vi "IP SNIFFER main vi.vi"() -> ()   [LabVIEW 2011]
doc: "This VI is an application to run through IP addresses starting at a specific IP and counting up by 1 however many times the user specifies."
uses:
  <vilib>/Utility/sysdir.llb/System Directory Type.ctl
panel:
  in  "Current IP":bool
  in  "Limit":bool
  out "Status":bool
  in  "Save results":bool
  out "Ping returns":T1(array[cluster])
  in  "stop scan":bool
  in  "scan":bool
  in  "Start IP Address (192.168.0.100)":string
  in  "Number of IPs to scan":i32 min=0 max=255 step=1
  in  "stop":bool
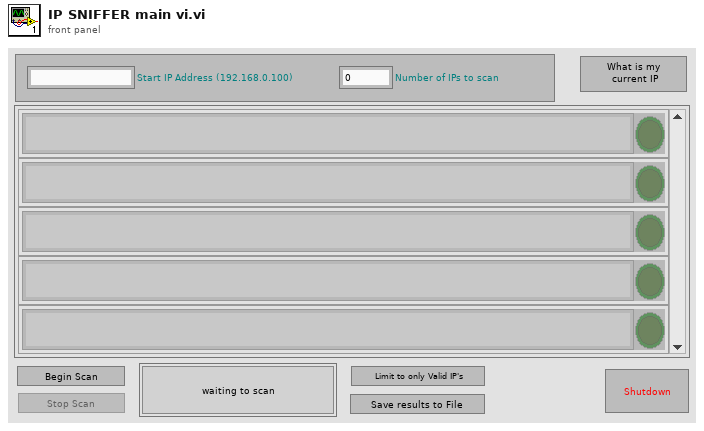
[diagram p1: front panel]
types:
  T1 = cluster{"Ping Status Return":string, "Valid IP (valid = true)":bool}[]
  T2 = cluster{"Ping Status Return":string, "Valid IP (valid = true)":bool}
  T3 = enum16{"open", "replace", "create", "open or create", "replace or create", "replace or create with confirmation"}
  T4 = typedef "System Directory Type.ctl" = i32
  T5 = enum8{"Enabled", "Disabled", "Disabled and Grayed Out"}
  T6 = enum32{"invalid app kind", "Development System", "Run Time System", "Student Edition", "Embedded LabVIEW", "Evaluation", "Custom"}
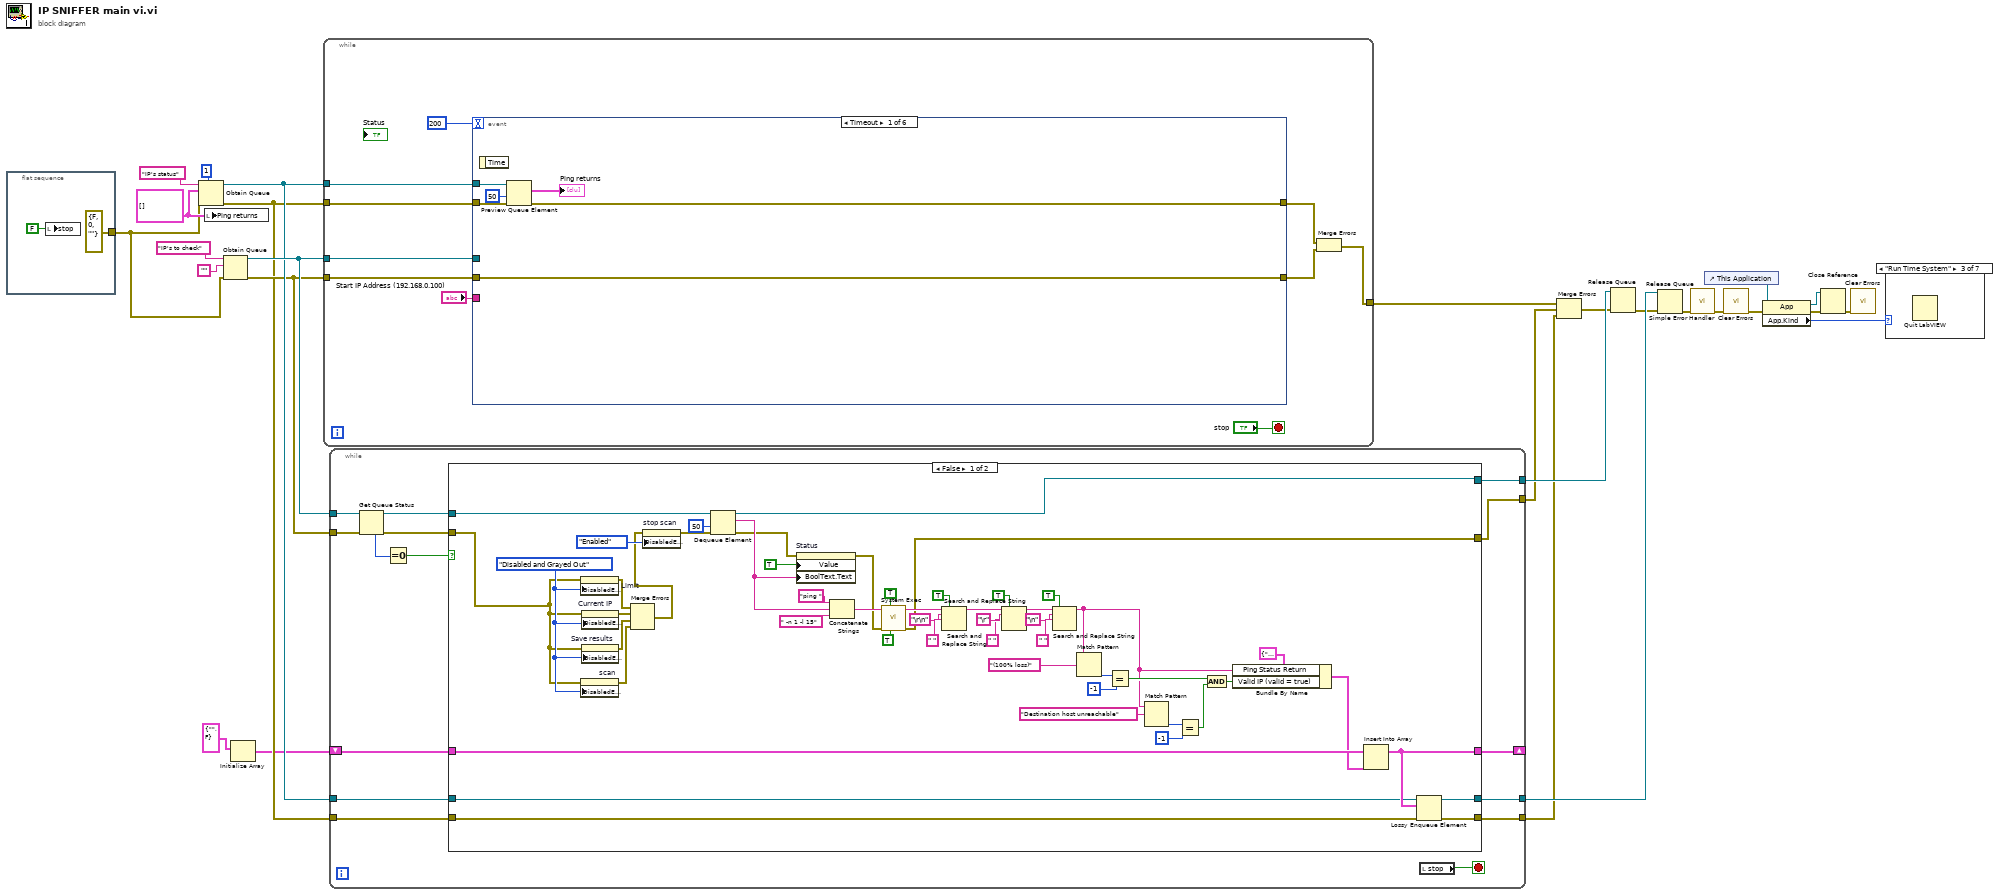
[diagram p0: block diagram]
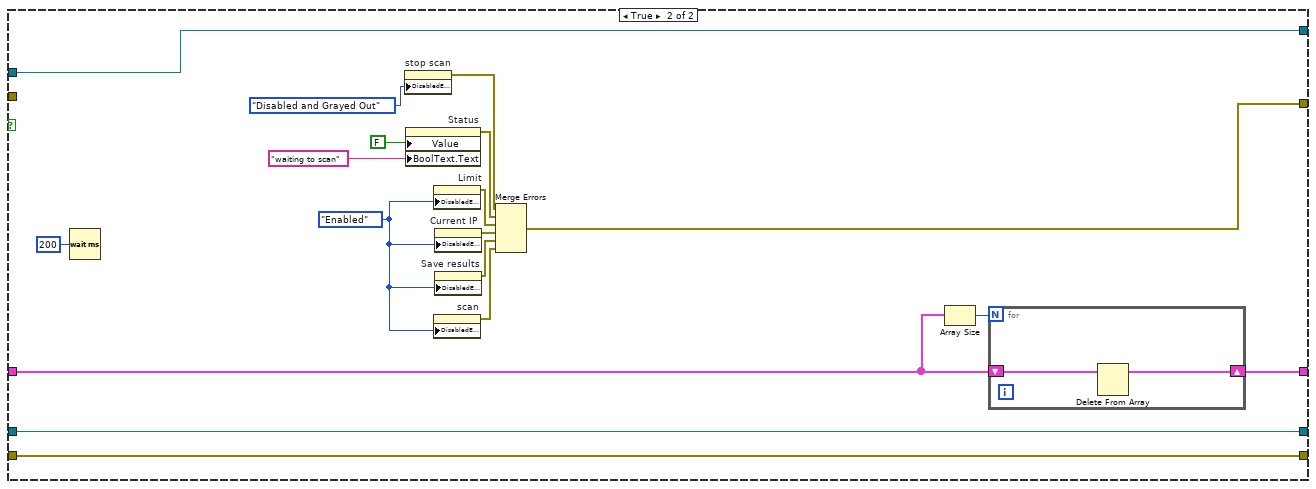
[diagram p2: hidden frame]
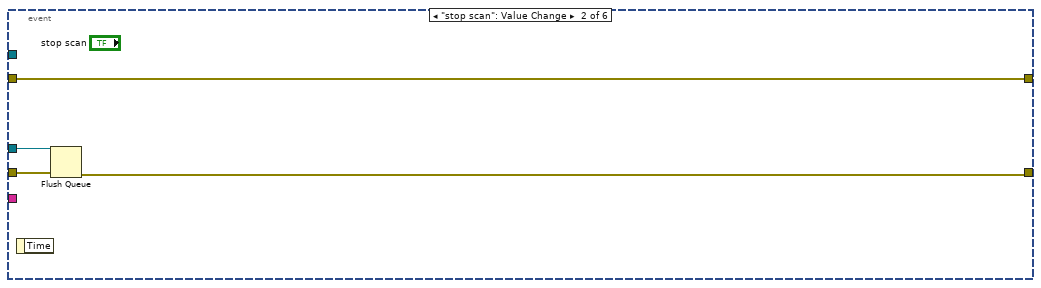
[diagram p9: hidden frame]
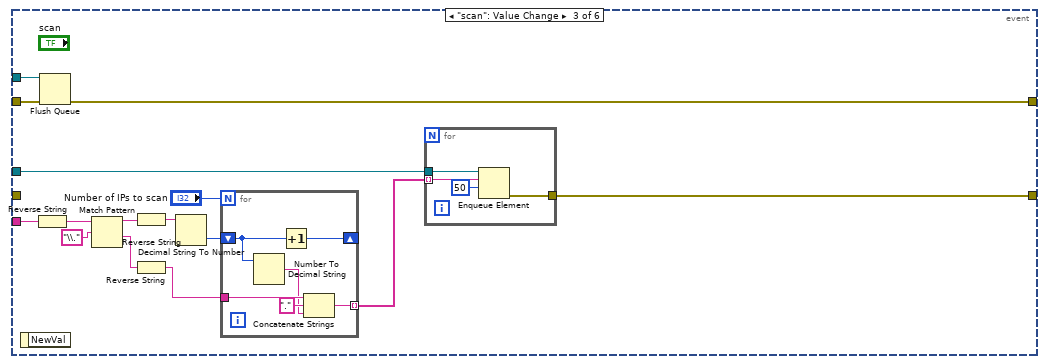
[diagram p10: hidden frame]
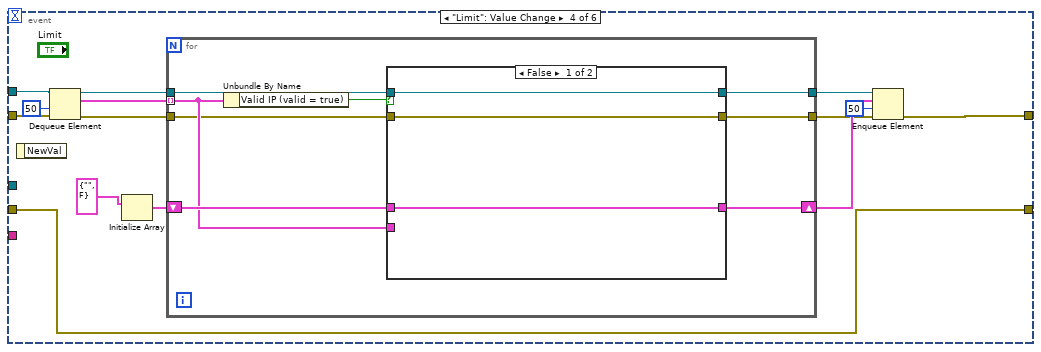
[diagram p11: hidden frame]
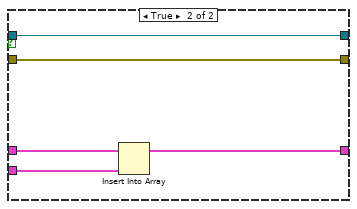
[diagram p12: hidden frame]
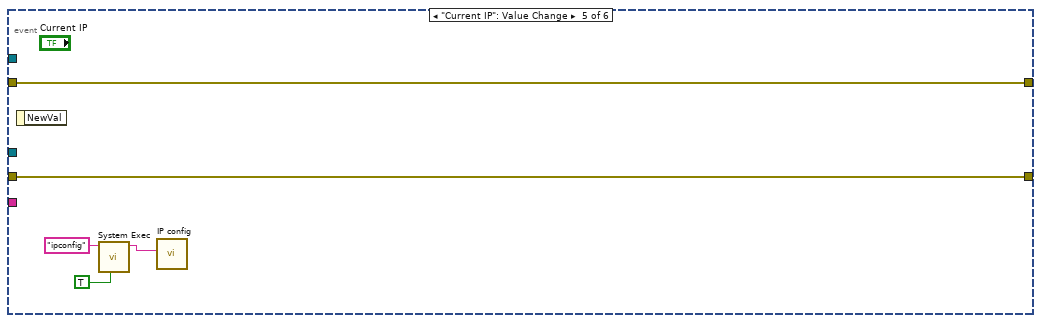
[diagram p13: hidden frame]
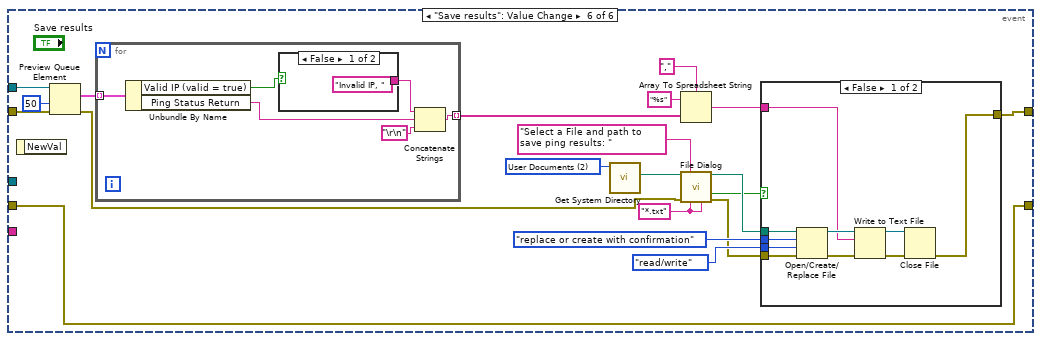
[diagram p14: hidden frame]
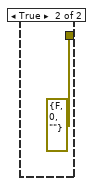
[diagram p15: hidden frame]
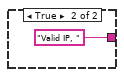
[diagram p16: hidden frame]
diagram:
  w15 = T1 [] ("Ping returns")
  n1 = flat-sequence {
    tunnel: [errorcluster {"status"=FALSE, "code"=0, "source"=""} ("error constant")] -> w6
    frame #0 {
      n2 = local write "stop"(FALSE ("stop")) -> ()
    }
  }
  n3 = Obtain Queue(max queue size (-1, unlimited)=1, name (unnamed)="IP's status", element data type=w15, error in (no error)=w6) -> (queue out=w14:refnum<queue>, error out=w12:errorcluster)  [unwired: 1 in, 1 out]
  n4 = local write "Ping returns"(w15) -> ()
  n5 = Obtain Queue(name (unnamed)="IP's to check", element data type="", error in (no error)=w6) -> (queue out=w19:refnum<queue>, error out=w13:errorcluster)  [unwired: 2 in, 1 out]
  n6 = Initialize Array(T2 {"Ping Status Return"="", "Valid IP (valid = true)"=FALSE}) -> (w10:T1)  [unwired: 1 in]
  n7 = while {
    tunnel: [w30] -> w25
    tunnel: w19 -> [w37]
    tunnel: w14 -> [w35]
    tunnel: w12 -> [w34]
    tunnel: w13 -> [w33]
    stop <- "stop" stop-if-true
    n8 = event shown="[0] Timeout" {
      selector: _ -> [_ _ _ _ _ _]
      dyn-events: _ -> [_ _ _ _ _ _]
      timeout: 200 -> [_ _ _ _ _ _]
      tunnel: "Start IP Address (192.168.0.100)" -> [_ _ w64 _ _ _]
      tunnel: w37 -> [_ w49 w55 _ _ _]
      tunnel: w35 -> [w44 _ w51 w86 _ w116]
      tunnel: w34 -> [w45 w46 w52 w81 w105 w115]
      tunnel: w33 -> [w42 w48 _ w77 w106 w111]
      tunnel: [w42 w47 w53 w77 w106 w111] -> w31
      tunnel: [w41 w46 w50 w78 w105 w112] -> w32
      event Timeout {
        n9 = event-data() -> ()  [unwired: 1 in, 1 out]
        n10 = Preview Queue Element(queue=w44, timeout in ms (-1)=50, error in (no error)=w45) -> (element=→"Ping returns":T1, error out=w41:errorcluster)  [unwired: 2 out]
      }
      event "stop scan": Value Change {
        n11 = event-data() -> ()  [unwired: 1 in, 1 out]
        n12 = Flush Queue(queue=w49, error in (no error)=w48) -> (error out=w47:errorcluster)  [unwired: 2 out]
      }
      event "scan": Value Change {
        n13 = event-data() -> ()  [unwired: 1 in, 1 out]
        n14 = Reverse String(1:w64) -> (0:w63:string)
        n15 = Flush Queue(queue=w51, error in (no error)=w52) -> (error out=w50:errorcluster)  [unwired: 2 out]
        n16 = Match Pattern(string=w63, regular expression="\\.") -> (before substring=w61:string, after substring=w59:string)  [unwired: 1 in, 2 out]
        n17 = Reverse String(1:w61) -> (0:w60:string)
        n18 = Reverse String(1:w59) -> (0:w58:string)
        n19 = Decimal String To Number(string=w60) -> (number=w56:i32)  [unwired: 2 in, 1 out]
        n20 = for {
          N: "Number of IPs to scan" -> [_]
          tunnel: [w74] -> w54 mode=indexing
          tunnel: w58 -> [w73]
          shift-right: [w70] -> _
          shift-left: w56 -> [w69]
          n21 = Number To Decimal String(number=w69) -> (decimal integer string=w71:string)  [unwired: 1 in]
          n22 = Increment(x=w69) -> (x+1=w70:i32)
          n23 = Concatenate Strings(w73, "." ("string"), w71) -> (w74:string)
        }
        n24 = for {
          tunnel: w55 -> [w68]
          tunnel: w54 -> [w67] mode=indexing
          tunnel: [w66] -> w53
          n25 = Enqueue Element(queue=w68, element=w67, timeout in ms (-1)=50) -> (error out=w66:errorcluster)  [unwired: 1 in, 2 out]
        }
      }
      event "Limit": Value Change {
        n26 = event-data() -> ()  [unwired: 1 in, 1 out]
        n27 = Dequeue Element(queue=w86, timeout in ms (-1)=50, error in (no error)=w81) -> (queue out=w84:refnum<queue>, element=w85:T1, error out=w80:errorcluster)  [unwired: 1 out]
        n28 = Initialize Array(T2 {"Ping Status Return"="", "Valid IP (valid = true)"=FALSE}) -> (w87:T1)  [unwired: 1 in]
        n29 = for {
          shift-right: [w94] -> w82
          shift-left: w87 -> [w95]
          tunnel: w85 -> [w93] mode=indexing
          tunnel: w84 -> [w92]
          tunnel: [w91] -> w83
          tunnel: w80 -> [w90]
          tunnel: [w89] -> w79
          n30 = Unbundle By Name(w93) -> ("Valid IP (valid = true)"=w96:bool)
          n31 = case shown="False" w96 {
            tunnel: w95 -> [w99 w103]
            tunnel: [w99 w104] -> w94
            tunnel: w93 -> [_ w102]
            tunnel: w92 -> [w98 w101]
            tunnel: [w98 w101] -> w91
            tunnel: w90 -> [w97 w100]
            tunnel: [w97 w100] -> w89
            frame False {
            }
            frame True {
              n32 = Insert Into Array(array=w103, new element=w102) -> (w104:T1)  [unwired: 1 in]
            }
          }
        }
        n33 = Enqueue Element(queue=w83, element=w82, timeout in ms (-1)=50, error in (no error)=w79) -> (error out=w78:errorcluster)  [unwired: 2 out]
      }
      event "Current IP": Value Change {
        n34 = event-data() -> ()  [unwired: 1 in, 1 out]
        n35 = call <vilib>:"System Exec.vi"("run minimized? (F)"=TRUE, "command line"="ipconfig") -> ("standard output"=w107:string)  [unwired: 6 in, 3 out]
        n36 = call "IP config"("Message"=w107) -> ()  [unwired: 9 in, 2 out]
      }
      event "Save results": Value Change {
        w120 = "*.txt" ("pattern (all files)")
        w123 = T4 2 items=["User Home"=0, "User Desktop"=1, "User Documents"=2, "User Application Data"=3, "User Preferences"=4, "User Temporary"=5, "Public Documents"=6, "Public Application Data"=7, "Public Preferences"=8, "Public Cache"=13, "System Core Libraries"=9, "System Installed Libraries"=10, "Application Files"=11, "Boot Volume Root"=12] ("system directory type")
        n37 = event-data() -> ()  [unwired: 1 in, 1 out]
        n38 = Preview Queue Element(queue=w116, timeout in ms (-1)=50, error in (no error)=w115) -> (element=w114:T1, error out=w113:errorcluster)  [unwired: 2 out]
        n39 = for {
          tunnel: [w143] -> w129 mode=indexing
          tunnel: w114 -> [w142] mode=indexing
          n40 = Unbundle By Name(w142) -> ("Valid IP (valid = true)"=w146:bool, "Ping Status Return"=w144:string)
          n41 = case shown="False" w146 {
            tunnel: ["Invalid IP, " "Valid IP, "] -> w145
            frame False {
            }
            frame True {
            }
          }
          n42 = Concatenate Strings(w145, w144, "\r\n") -> (w143:string)
        }
        n43 = call <vilib>:"Get System Directory.vi"("system directory type"=w123) -> ("system directory"=w122:path)  [unwired: 10 in]
        n44 = Array To Spreadsheet String(delimiter (Tab)=",", array=w129, 3:"%s" ("format string")) -> (spreadsheet string=w124:string)
        n45 = call "File Dialog"("start path"=w122, "prompt"="Select a File and path to save ping results: ", "error in"=w113, "pattern (all files)"=w120, "pattern label"=w120) -> ("selected path"=w119:path, "cancelled"=w117:bool, "error out"=w118:errorcluster)  [unwired: 7 in, 1 out]
        n46 = case shown="False" w117 {
          tunnel: T3."replace or create with confirmation" ("operation (0:open)") -> [w139 _]
          tunnel: enum16{"read/write", "read-only", "write-only"}."read/write" ("access (0:read/write)") -> [w138 _]
          tunnel: w124 -> [w135 _]
          tunnel: w119 -> [w132 _]
          tunnel: w118 -> [w131 _]
          tunnel: [w130 errorcluster {"status"=FALSE, "code"=0, "source"=""} ("error out")] -> w112
          frame False {
            n47 = Open/Create/Replace File(file path (use dialog)=w132, error in=w131, operation (0:open)=w139, access (0:read/write)=w138) -> (refnum out=w137:refnum<file>, error out=w136:errorcluster)  [unwired: 2 in, 1 out]
            n48 = Write to Text File(file (use dialog)=w137, text=w135, error in=w136) -> (refnum out=w133:refnum<file>, error out=w134:errorcluster)  [unwired: 1 in, 1 out]
            n49 = Close File(refnum=w133, error in=w134) -> (error out=w130:errorcluster)  [unwired: 1 out]
          }
          frame True {
          }
        }
      }
    }
    n50 = Merge Errors(w32, w31) -> (w30:errorcluster)
  }
  n51 = while {
    tunnel: w19 -> [w163]
    tunnel: [w157] -> w18
    tunnel: [w156] -> w5
    tunnel: w14 -> [w155]
    tunnel: w13 -> [w154]
    tunnel: w12 -> [w153]
    shift-right: [w151] -> _
    shift-left: w10 -> [w152]
    tunnel: [w150] -> w9
    tunnel: [w149] -> w4
    stop <- w158 stop-if-true
    n52 = Get Queue Status(queue=w163, error in (no error)=w154) -> (queue out=w160:refnum<queue>, error out=w159:errorcluster, # elements in queue=w162:i32)  [unwired: 1 in, 5 out]
    n53 = Equal To 0?(x=w162) -> (x = 0?=w161:bool)
    n54 = case shown="False" w161 {
      tunnel: w160 -> [w181 w222]
      tunnel: w159 -> [w166 _]
      tunnel: [w167 w223] -> w156
      tunnel: [w175 w222] -> w157
      tunnel: w155 -> [w171 w221]
      tunnel: w153 -> [w164 w220]
      tunnel: w152 -> [w174 w217]
      tunnel: [w172 w219] -> w151
      tunnel: [w170 w221] -> w150
      tunnel: [w169 w220] -> w149
      frame False {
        w186 = T5."Disabled and Grayed Out" ("Disabled")
        n55 = property on="Limit" class="Bool"(error in=w166, "DisabledEnum"=w186) -> (error out=w182:errorcluster)  [unwired: 1 in, 1 out]
        n56 = property on="scan" class="Bool"(error in=w166, "DisabledEnum"=w186) -> (error out=w185:errorcluster)  [unwired: 1 in, 1 out]
        n57 = property on="Current IP" class="Bool"(error in=w166, "DisabledEnum"=w186) -> (error out=w183:errorcluster)  [unwired: 1 in, 1 out]
        n58 = property on="Save results" class="Bool"(error in=w166, "DisabledEnum"=w186) -> (error out=w184:errorcluster)  [unwired: 1 in, 1 out]
        n59 = Merge Errors(w182, w183, w184, w185) -> (w165:errorcluster)
        n60 = property on="stop scan" class="Bool"(error in=w165, "DisabledEnum"=T5."Enabled" ("Disabled")) -> (error out=w178:errorcluster)  [unwired: 1 in, 1 out]
        n61 = Dequeue Element(queue=w181, timeout in ms (-1)=50, error in (no error)=w178) -> (queue out=w175:refnum<queue>, element=w180:string, error out=w177:errorcluster)  [unwired: 1 out]
        n62 = property on="Status" class="Bool (strict)"(error in=w177, "Value"=TRUE ("Status"), "BoolText.Text"=w180) -> (error out=w176:errorcluster)  [unwired: 1 in, 1 out]
        n63 = Concatenate Strings("ping " ("string"), w180, " -n 1 -l 15" ("string")) -> (w189:string)
        n64 = call <vilib>:"System Exec.vi"("run minimized? (F)"=TRUE, "wait until completion? (T)"=TRUE, "error in (no error)"=w176, "command line"=w189) -> ("error out"=w167:errorcluster, "standard output"=w191:string)  [unwired: 4 in, 2 out]
        n65 = Search and Replace String(replace all?=TRUE ("replace all? (F)"), input string=w191, search string="\r\n", replace string=" " ("replace string (\"\")")) -> (result string=w201:string)  [unwired: 4 in, 3 out]
        n66 = Search and Replace String(replace all?=TRUE ("replace all? (F)"), input string=w201, search string="\r", replace string=" " ("replace string (\"\")")) -> (result string=w200:string)  [unwired: 4 in, 3 out]
        n67 = Search and Replace String(replace all?=TRUE ("replace all? (F)"), input string=w200, search string="\n", replace string=" " ("replace string (\"\")")) -> (result string=w207:string)  [unwired: 4 in, 3 out]
        n68 = Match Pattern(string=w207, regular expression="(100% loss)") -> (offset past match=w203:i32)  [unwired: 1 in, 3 out]
        n69 = Equal?(x=w203, y=-1) -> (x = y?=w210:bool)
        n70 = Match Pattern(string=w207, regular expression="Destination host unreachable") -> (offset past match=w206:i32)  [unwired: 1 in, 3 out]
        n71 = Equal?(x=w206, y=-1) -> (x = y?=w209:bool)
        n72 = And(x=w210, y=w209) -> (x .and. y?=w211:bool)
        n73 = Bundle By Name(cluster=T2 {"Ping Status Return"="  Pinging 192.168.0.100 with 32 bytes of data:    Request timed out.  Request timed out.  Request timed out.  Request timed out.    Ping statistics for 192.168.0.100:      Packets: Sent = 4, Received = 0, Lost = 4 ", "Valid IP (valid = true)"=FALSE}, "Ping Status Return"=w207, "Valid IP (valid = true)"=w211) -> (w173:T2)
        n74 = Insert Into Array(array=w174, new element=w173) -> (w172:T1)  [unwired: 1 in]
        n75 = Lossy Enqueue Element(queue=w171, element=w172, error in (no error)=w164) -> (queue out=w170:refnum<queue>, error out=w169:errorcluster)  [unwired: 2 out]
      }
      frame True {
        w226 = T5."Enabled" ("Disabled")
        n76 = Wait (ms)(milliseconds to wait=u32 200) -> ()  [unwired: 1 out]
        n77 = property on="stop scan" class="Bool"("DisabledEnum"=T5."Disabled and Grayed Out" ("Disabled")) -> (error out=w232:errorcluster)  [unwired: 2 in, 1 out]
        n78 = property on="Status" class="Bool (strict)"("Value"=FALSE ("Status"), "BoolText.Text"="waiting to scan" ("Boolean Text.Text")) -> (error out=w227:errorcluster)  [unwired: 2 in, 1 out]
        n79 = property on="Limit" class="Bool"("DisabledEnum"=w226) -> (error out=w228:errorcluster)  [unwired: 2 in, 1 out]
        n80 = property on="scan" class="Bool"("DisabledEnum"=w226) -> (error out=w231:errorcluster)  [unwired: 2 in, 1 out]
        n81 = property on="Current IP" class="Bool"("DisabledEnum"=w226) -> (error out=w229:errorcluster)  [unwired: 2 in, 1 out]
        n82 = property on="Save results" class="Bool"("DisabledEnum"=w226) -> (error out=w230:errorcluster)  [unwired: 2 in, 1 out]
        n83 = Merge Errors(w232, w227, w228, w229, w230, w231) -> (w223:errorcluster)
        n84 = Array Size(array=w217) -> (size(s)=w218:i32)
        n85 = for {
          N: w218 -> [_]
          shift-right: [w234] -> w219
          shift-left: w217 -> [w235]
          n86 = Delete From Array(array=w235) -> (array with subset deleted=w234:T1)  [unwired: 2 in, 1 out]
        }
      }
    }
    n87 = local read "stop"() -> (w158:bool)
  }
  n88 = Merge Errors(w25, w5, w4) -> (w3:errorcluster)
  n89 = Release Queue(queue=w18, error in (no error)=w3) -> (error out=w2:errorcluster)  [unwired: 1 in, 2 out]
  n90 = Release Queue(queue=w9, error in (no error)=w2) -> (error out=w1:errorcluster)  [unwired: 1 in, 2 out]
  n91 = call <vilib>:"Simple Error Handler.vi"("error in (no error)"=w1) -> ("error out"=w8:errorcluster)  [unwired: 4 in, 4 out]
  n92 = control-ref of="This Application"() -> (w27:refnum<vi>)
  n93 = call <vilib>:"Clear Errors.vi"("error in (no error)"=w8) -> ("error out"=w7:errorcluster)  [unwired: 6 in]
  n94 = property class="App"(reference=w27, error in=w7) -> (reference out=w23:refnum<vi>, error out=w24:errorcluster, "App.Kind"=w26:T6)
  n95 = Close Reference(reference=w23, error in (no error)=w24) -> (error out=w22:errorcluster)
  n96 = call <vilib>:"Clear Errors.vi"("error in (no error)"=w22) -> ()  [unwired: 6 in, 1 out]
  n97 = case shown="\"Run Time System\"" w26 {
    frame "invalid app kind", Default {
    }
    frame "Development System" {
    }
    frame "Run Time System" {
      n98 = Quit LabVIEW() -> ()  [unwired: 1 in]
    }
    frame "Student Edition" {
    }
    frame "Embedded LabVIEW" {
    }
    frame "Evaluation" {
    }
    frame "Custom" {
    }
  }
